vi "Teleop.vi"(10 "Match Info":T1={"Autonomous Elapsed Seconds"=0.0, "TeleOp Elapsed Seconds"=0.0, "Disabled Elapsed Seconds"=0.0, "Visited Autonomous"=FALSE, "Visited TeleOp"=FALSE, "Visited Disabled"=FALSE, "Autonomous Settings"={"Autonomous Style"=enum."Independent", "VI Refnum"=refnum}}, 11 "Call Context":T2) -> ()   [LabVIEW 2012]
doc: "This VI is called for each TeleOp packet received from the DS where the robot is not disabled. It is often used to read from the joysticks and update I/O or to update setpoints for timed control loops. It should complete and return within 20 milliseconds or it may miss DS packets."
uses:
  <vilib>/Rock Robotics/WPI/DriverStation/WPI_DriverStationDerivedRobotMode.ctl
  <vilib>/Rock Robotics/WPI/DriverStation/WPI_DriverStationMatch Info.ctl
  Robot Global Data.vi
  <vilib>/Rock Robotics/WPI/Joystick/WPI_JoystickGetSetRefNum.vi
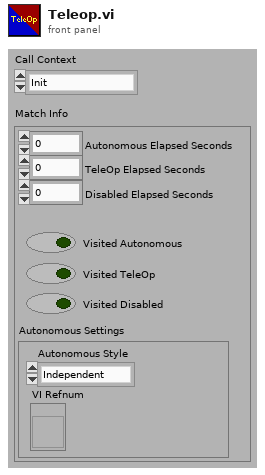
[diagram p1: front panel]
types:
  T1 = typedef "WPI_DriverStationMatch Info.ctl" = cluster{"Autonomous Elapsed Seconds":dbl, "TeleOp Elapsed Seconds":dbl, "Disabled Elapsed Seconds":dbl, "Visited Autonomous":bool, "Visited TeleOp":bool, "Visited Disabled":bool, "Autonomous Settings":cluster{"Autonomous Style":enum16{"Iterative", "Independent"}, "VI Refnum":refnum<vi>}}
  T2 = typedef "WPI_DriverStationDerivedRobotMode.ctl" = enum16{"Init", "Execute", "Stop"}
  T3 = typedef "WPI_JoystickDevRef.ctl" = cluster{"Device":T4}
  T4 = typedef "WPI_JoystickDeviceEnum.ctl" = enum16{"USB 1", "USB 2", "USB 3", "USB 4", "Kinect 1", "Kinect 2"}
  T5 = typedef "WPI_JoystickButtonState.ctl" = cluster{"Button 1":bool, "Button 2":bool, "Button 3":bool, "Button 4":bool, "Button 5":bool, "Button 6":bool, "Button 7":bool, "Button 8":bool, "Button 9":bool, "Button 10":bool, "Button 11":bool, "Button 12":bool}
  T6 = cluster{"axis 1 (x)":dbl, "axis 2 (y)":dbl, "axis 3 (throttle)":dbl, "axis 4":dbl, "axis 5":dbl, "axis 6":dbl}
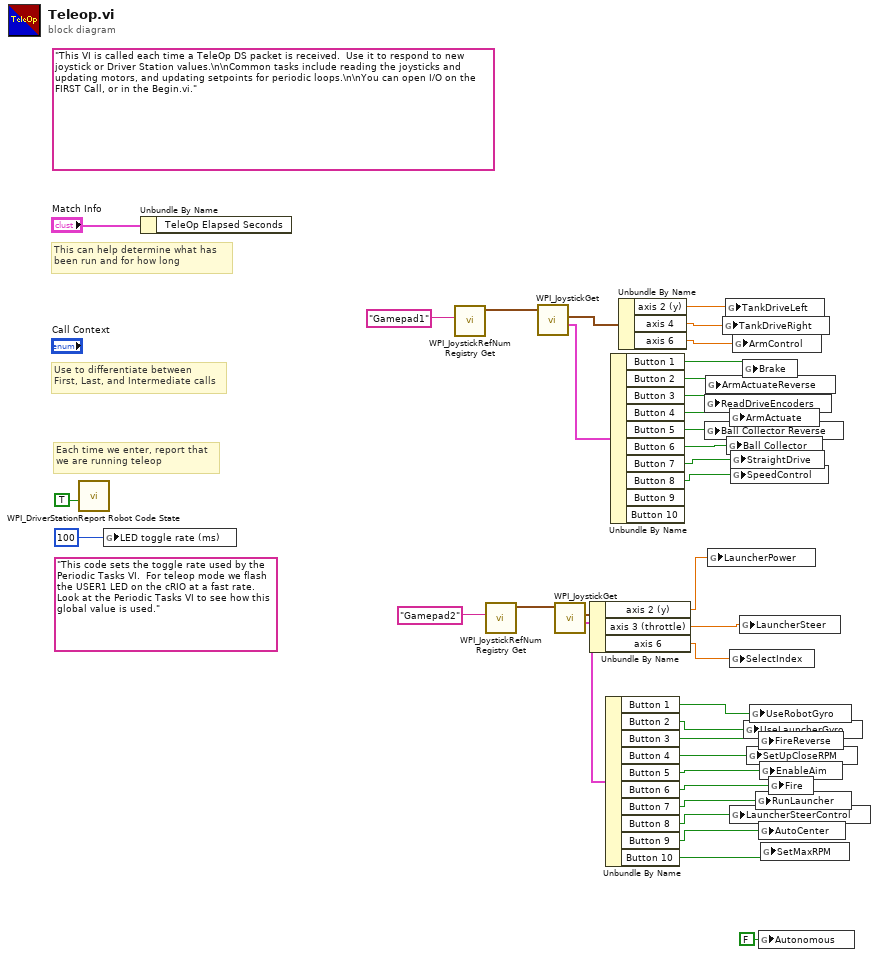
[diagram p0: block diagram]
diagram:
  (unwired) "This code sets the toggle rate used by the Periodic Tasks VI.  For teleop mode we flash the USER1 LED on the cRIO at a fast rate.  Look at the Periodic Tasks VI to see how this global value is used."
  (unwired) "This VI is called each time a TeleOp DS packet is received.  Use it to respond to new joystick or Driver Station values.\n\nCommon tasks include reading the joysticks and updating motors, and updating setpoints for periodic loops.\n\nYou can open I/O on the FIRST Call, or in the Begin.vi."
  # "Each time we enter, report that\nwe are running teleop"
  # "Use to differentiate between\nFirst, Last, and Intermediate calls"
  # "This can help determine what has\nbeen run and for how long"
  n1 = call <vilib>:"WPI_DriverStationReport Robot Code State.vi"("TeleOp"=TRUE ("Autonomous")) -> ()  [unwired: 10 in, 1 out]
  n2 = global write "Robot Global Data.vi" "LED toggle rate (ms)"(u32 100 ("LED ms toggle rate")) -> ()
  n3 = Unbundle By Name("Match Info") -> ()  [unwired: 1 out]
  n4 = call <vilib>:"WPI_JoystickRefNum Registry Get.vi"("refnum name"="Gamepad1") -> ("JoystickDevRef"=w32:T3)  [unwired: 9 in, 1 out]
  n5 = call <vilib>:"WPI_JoystickRefNum Registry Get.vi"("refnum name"="Gamepad2") -> ("JoystickDevRef"=w23:T3)  [unwired: 9 in, 1 out]
  n6 = call <vilib>:"WPI_JoystickGet.vi"("JoystickDevRef"=w32) -> ("Buttons"=w28:T5, "Axes"=w31:T6)  [unwired: 4 in, 1 out]
  n7 = call <vilib>:"WPI_JoystickGet.vi"("JoystickDevRef"=w23) -> ("Buttons"=w22:T5, "Axes"=w18:T6)  [unwired: 4 in, 1 out]
  n8 = Unbundle By Name(w18) -> ("axis 2 (y)"=w17:dbl, "axis 3 (throttle)"=w16:dbl, "axis 6"=w7:dbl)
  n9 = Unbundle By Name(w22) -> ("Button 1"=w11:bool, "Button 2"=w10:bool, "Button 3"=w8:bool, "Button 4"=w6:bool, "Button 5"=w19:bool, "Button 6"=w20:bool, "Button 7"=w21:bool, "Button 8"=w4:bool, "Button 9"=w5:bool, "Button 10"=w12:bool)
  n10 = Unbundle By Name(w28) -> ("Button 1"=w14:bool, "Button 2"=w1:bool, "Button 3"=w3:bool, "Button 4"=w2:bool, "Button 5"=w15:bool, "Button 6"=w27:bool, "Button 7"=w25:bool, "Button 8"=w26:bool)  [unwired: 2 out]
  n11 = Unbundle By Name(w31) -> ("axis 2 (y)"=w30:dbl, "axis 4"=w29:dbl, "axis 6"=w9:dbl)
  n12 = global write "Robot Global Data.vi" "ReadDriveEncoders"(w3) -> ()
  n13 = global write "Robot Global Data.vi" "Ball Collector Reverse"(w15) -> ()
  n14 = global write "Robot Global Data.vi" "ArmActuateReverse"(w1) -> ()
  n15 = global write "Robot Global Data.vi" "LauncherPower"(w17) -> ()
  n16 = global write "Robot Global Data.vi" "TankDriveRight"(w29) -> ()
  n17 = global write "Robot Global Data.vi" "TankDriveLeft"(w30) -> ()
  n18 = global write "Robot Global Data.vi" "Ball Collector"(w27) -> ()
  n19 = global write "Robot Global Data.vi" "ArmActuate"(w2) -> ()
  n20 = global write "Robot Global Data.vi" "SelectIndex"(w7) -> ()
  n21 = global write "Robot Global Data.vi" "LauncherSteerControl"(w4) -> ()
  n22 = global write "Robot Global Data.vi" "StraightDrive"(w25) -> ()
  n23 = global write "Robot Global Data.vi" "SpeedControl"(w26) -> ()
  n24 = global write "Robot Global Data.vi" "ArmControl"(w9) -> ()
  n25 = global write "Robot Global Data.vi" "LauncherSteer"(w16) -> ()
  n26 = global write "Robot Global Data.vi" "Brake"(w14) -> ()
  n27 = global write "Robot Global Data.vi" "UseLauncherGyro"(w10) -> ()
  n28 = global write "Robot Global Data.vi" "SetUpCloseRPM"(w6) -> ()
  n29 = global write "Robot Global Data.vi" "UseRobotGyro"(w11) -> ()
  n30 = global write "Robot Global Data.vi" "RunLauncher"(w21) -> ()
  n31 = global write "Robot Global Data.vi" "FireReverse"(w8) -> ()
  n32 = global write "Robot Global Data.vi" "AutoCenter"(w5) -> ()
  n33 = global write "Robot Global Data.vi" "Autonomous"(FALSE ("Autonomous")) -> ()
  n34 = global write "Robot Global Data.vi" "EnableAim"(w19) -> ()
  n35 = global write "Robot Global Data.vi" "SetMaxRPM"(w12) -> ()
  n36 = global write "Robot Global Data.vi" "Fire"(w20) -> ()
